vi "STM Read Meta Data (TCP Clst).vi"(6 "Options":T3={"Ignore Timeout Error"=TRUE, "timeout ms (1000)"=1000}, 8 "error in":errorcluster, 11 "Connection Info In":T1) -> (0 "error out":errorcluster, 1 "Meta data":T2[](array[typedef]), 3 "Connection Info Out":T1)   [LabVIEW 2015, in "Diagnostics Addon Engine.lvlib"]
doc: "This VI reads the meta data information from a remote computer. Use this VI to retrieve the variable names and types that a remote computer exports.\n\nThis VI parses the data and returns a cluster containing the meta data information."
uses:
  Diagnostics Addon Engine.lvlib
  _SubVIs/stm_MetaDataElement.ctl
  stm_TCP Read Options.ctl
  stm_TCP Connection Info.ctl
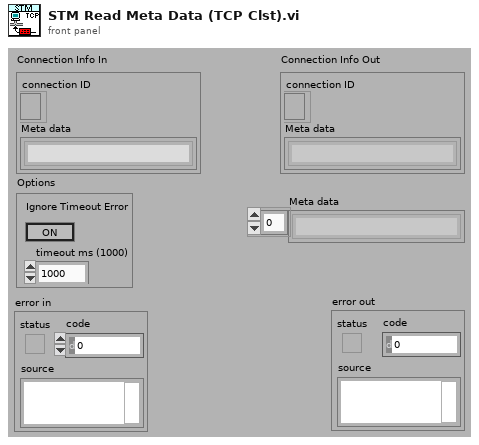
[diagram p1: front panel]
types:
  T1 = typedef "Diagnostics Addon Engine.lvlib/stm_TCP Connection Info.ctl" = cluster{"connection ID":refnum<k5>, "Meta data":T2[]}
  T2 = typedef "Diagnostics Addon Engine.lvlib/stm_MetaDataElement.ctl" = string
  T3 = typedef "Diagnostics Addon Engine.lvlib/stm_TCP Read Options.ctl" = cluster{"Ignore Timeout Error":bool, "timeout ms (1000)":i32}
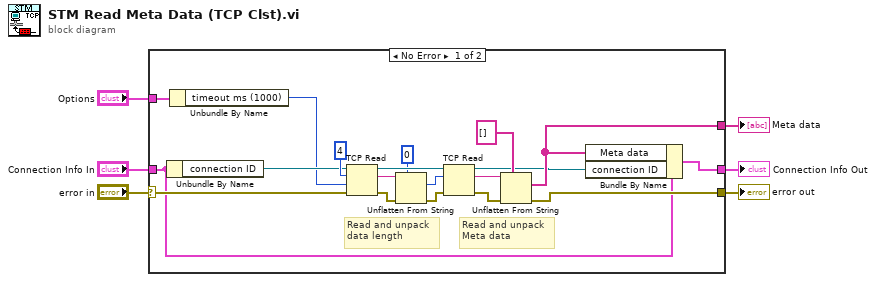
[diagram p0: block diagram]
diagram:
  n1 = case shown="No Error" "error in" {
    selector: "error in" -> [w14 w27]
    tunnel: [w13 _] -> w6
    tunnel: [w25 w27] -> w5
    tunnel: [w11 w26] -> w1
    tunnel: "Options" -> [w10 _]
    tunnel: "Connection Info In" -> [w7 w26]
    frame No Error {
      # "Read and unpack\nMeta data"
      # "Read and unpack\ndata length"
      n2 = Unbundle By Name(w7) -> ("connection ID"=w9:refnum<k5>)
      n3 = Unbundle By Name(w10) -> ("timeout ms (1000)"=w8:i32)
      n4 = TCP Read(connection ID=w9, bytes to read=4, error in (no error)=w14, 9:w8) -> (connection ID out=w22:refnum<k5>, data out=w19:string, error out=w15:errorcluster)  [unwired: 1 out]
      n5 = Unflatten From String(type=0 ("bytes to read"), binary string=w19, error in (no error)=w15) -> (value=w16:i32, error out=w17:errorcluster)  [unwired: 3 out]
      n6 = TCP Read(connection ID=w22, bytes to read=w16, error in (no error)=w17) -> (connection ID out=w12:refnum<k5>, data out=w21:string, error out=w20:errorcluster)  [unwired: 2 out]
      n7 = Unflatten From String(type=T2[] [] ("Meta data"), binary string=w21, error in (no error)=w20) -> (value=w13:T2[], error out=w25:errorcluster)  [unwired: 3 out]
      n8 = Bundle By Name(cluster=w7, "Meta data"=w13, "connection ID"=w12) -> (w11:T1)
    }
    frame Error {
    }
  }
  "Meta data" <- w6
  "error out" <- w5
  "Connection Info Out" <- w1
